vi "Shooter_WinchNoPID.vi"(6 "PickStartPos":dbl, 7 "WinchFiredPos":dbl=3.3, 8 "Winch Pot Location":dbl, 9 "WinchPower":dbl=0.75, 10 "selectedCase":i32, 11 "SetPointArray":dbl[](array[numeric])=[1.0, 2.0, 3.0]) -> (0 "isThere?":bool, 3 "Winch Motor Power Out":dbl)   [LabVIEW 2013]
panel:
  in  "slow power":dbl=0.45 format="%#_13g"
  out "Winch Desired Location":dbl
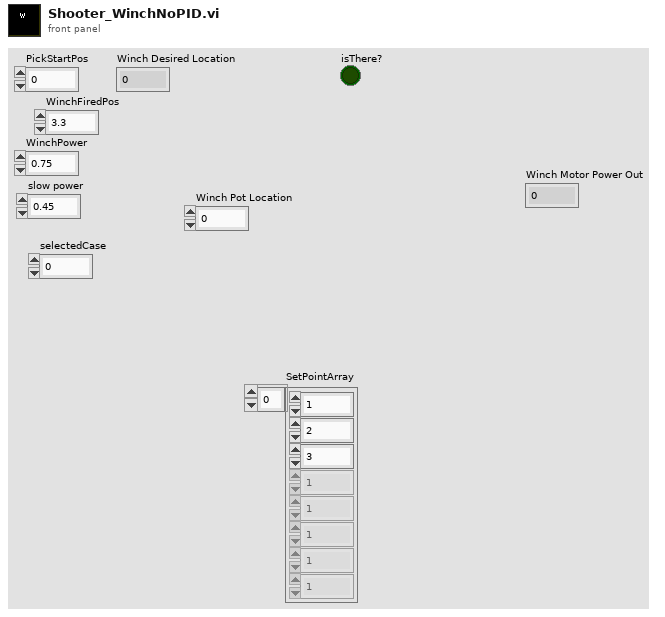
[diagram p1: front panel]
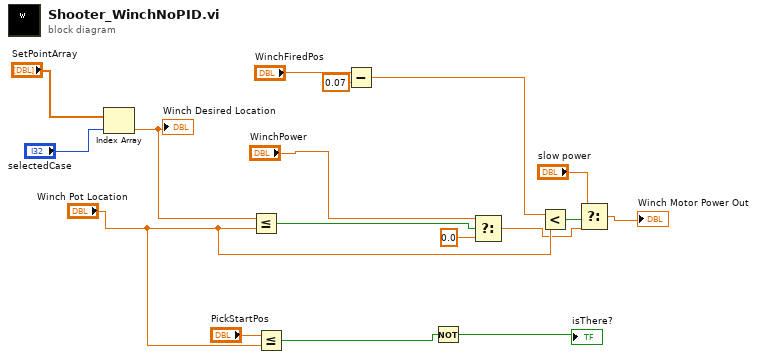
[diagram p0: block diagram]
diagram:
  n1 = Index Array(array="SetPointArray", index="selectedCase") -> (element=w14:dbl)
  "Winch Desired Location" <- w14
  n2 = Less Or Equal?(x=w14, y="Winch Pot Location") -> (x <= y?=w13:bool)
  n3 = Less Or Equal?(x="PickStartPos", y="Winch Pot Location") -> (x <= y?=w12:bool)
  n4 = Subtract(x="WinchFiredPos", y=0.07) -> (x-y=w4:dbl)
  n5 = Not(x=w12) -> (.not. x?=→"isThere?":bool)
  n6 = Select(t="WinchPower", s=w13, f=0.0) -> (s? t:f=w9:dbl)
  n7 = Less?(x=w4, y="Winch Pot Location") -> (x < y?=w8:bool)
  n8 = Select(t="slow power", s=w8, f=w9) -> (s? t:f=→"Winch Motor Power Out":dbl)
